vi "ECT in Run on Parametric.vi"(8 "Error In":errorcluster, 9 "ECT Parameters":T1={"MS to Spin Time"=0, "Target Fill Time"=238, "MS to Agitate Time"=0, "MS to Spin before Spin Time "=0, "Adaptive Drain Time"=180, "Coast to 0 Time"=60}, 10 "Option Selection":T2={"Soil Level"=enum."Normal", "Warm Rinse"=enum."Disable", "Fabric Softener"=enum."Disable", "Extra Rinse"=enum."Disable", "Soak"=enum."Level 0", "Stain"=enum."Off", "Spin"=enum."Normal Spin", "Load Size"=enum."Precise Fill", "Dry Load Size"=enum."65535", "Load Type"=enum."Unknown", "Deep Fill"=enum."Off"}, 11 "GEA2 Reference In":refnum<k24>) -> (0 "Error Out":errorcluster, 1 "Pass/Fail?":bool, 2 "Report Text":string, 3 "GEA2 Reference Out":refnum<k24>, 4 "Actual ECT (sec)":u16, 5 "Expected ECT (sec)":u16)   [LabVIEW 2016, in "Centauro.lvlib"]
uses:
  Projects/Centauro.lvlib
  Common/LabVIEW GEA2 Toolkit/LabVIEW_GEA2_Toolkit.lvlibp/type defs/Source_Destination.ctl
  Common/LabVIEW GEA2 Toolkit/LabVIEW_GEA2_Toolkit.lvlibp
  Valew Common/type defs/Encoder Position.ctl
  Common/LabVIEW GEA2 Toolkit/LabVIEW_GEA2_Toolkit.lvlibp/type defs/Data Type.ctl
  Common/LabVIEW GEA2 Toolkit/LabVIEW_GEA2_Toolkit.lvlibp/type defs/ERD Write Data In.ctl
  Valew Common/type defs/UI Buttons.ctl
  Common/LabVIEW GEA2 Toolkit/LabVIEW_GEA2_Toolkit.lvlibp/type defs/ERD Read Data In.ctl
  Q:/Common/DLLs/GEA3/GeaCommunication.dll
  Common/DLLs/GEA3/GeaCommunication.dll
  Controls/Options.ctl
  Controls/ECT Parameters.ctl
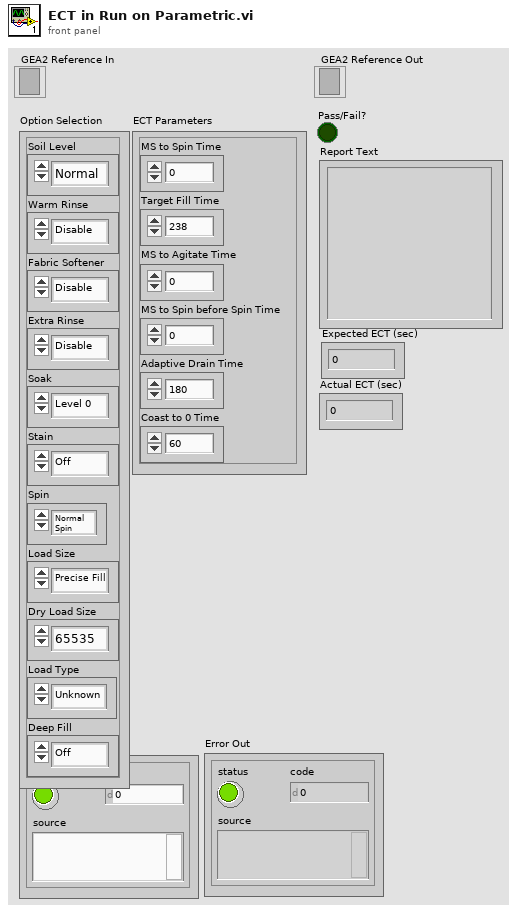
[diagram p1: front panel]
types:
  T1 = typedef "Centauro.lvlib/ECT Parameters.ctl" = cluster{"MS to Spin Time":u16, "Target Fill Time":u16, "MS to Agitate Time":u16, "MS to Spin before Spin Time ":u16, "Adaptive Drain Time":u16, "Coast to 0 Time":u16}
  T2 = typedef "Centauro.lvlib/Options.ctl" = cluster{"Soil Level":enum8{"Ex Light", "Light", "Normal", "Heavy", "Ex Heavy"}, "Warm Rinse":enum8{"Disable", "Enable"}, "Fabric Softener":enum16{"Disable", "Enable"}, "Extra Rinse":enum8{"Disable", "Enable"}, "Soak":enum8{"Level 0", "Level 1", "Level 2", "Level 3", "Level 4"}, "Stain":enum8{"Off", "Tomato", "Wine", "Blood", "Grass", "Dirt"}, "Spin":enum16{"No Spin", "Normal Spin", "More Spin", "Max Spin"}, "Load Size":enum8{"Small", "Medium", "Large", "Super", "Precise Fill", "Super Plus"}, "Dry Load Size":enum16{"128", "256", "384", "5AA", "6A4", "834", "65535"}, "Load Type":enum8{"Unknown", "Cotton", "Synthetic", "Mixed", "Wet", "Low Flow", "Small", "Medium", "Large", "Super", "Super Plus", "Max"}, "Deep Fill":enum8{"Off", "Incremental Fill", "Max Fill"}}
  T3 = typedef "LabVIEW_GEA2_Toolkit.lvlibp/Source_Destination.ctl" = cluster{"Source":u8, "Destination":u8}
  T4 = typedef "LabVIEW_GEA2_Toolkit.lvlibp/ERD Read Data In.ctl" = cluster{"ERD Number":u16, "Data Type":T5}
  T5 = typedef "LabVIEW_GEA2_Toolkit.lvlibp/Data Type.ctl" = enum16{"string", "boolean", "uint8_t", "uint16_t", "uint32_t", "uint64_t", "int8_t", "int16_t", "int32_t", "int64_t"}
  T6 = typedef "Centauro.lvlib/UI Buttons.ctl" = enum16{"Switch Off", "SW201 - My Cycle", "SW202 - Delay Wash", "SW203 - Extra Rinse", "SW204 - Signal / Volume", "SW205 - Spin", "SW206 - Deep Rinse / Fab Soft", "SW207 - Soil", "SW208 - Auto Soak", "SW209 - Temp", "SW210 - Warm Rinse", "SW211 - Deep Fill", "SW212 - Stain Remover", "SW213 - Power", "SW222 - Control Lock", "SW214 - Start / Pause", "SW301 - Start/Pause LE", "SW302 - Option Button LE", "SW201/212 - Bulk Flush"}
  T7 = typedef "LabVIEW_GEA2_Toolkit.lvlibp/ERD Write Data In.ctl" = cluster{"ERD Number":u16, "Data Type":T5, "Data":string}
  T8 = typedef "Centauro.lvlib/Encoder Position.ctl" = enum16{"Position 0", "Position 1", "Position 2", "Position 3", "Position 4", "Position 5", "Position 6", "Position 7", "Position 8", "Position 9", "Position 10", "Position 11", "Position 12", "Position 13", "Clear / Reset"}
  T9 = typedef "LabVIEW_GEA2_Toolkit.lvlibp/ERD Read Data Out.ctl" = cluster{"ERD Number":u16, "Data":string}
  T10 = typedef "Centauro.lvlib/ECT.ctl" = cluster{"MS to Agitate Time":u16, "Adaptive Drain Time":u16, "Coast to 0 Time":u16, "Agitate Time":u16, "Warm Rinse Time":u16, "FS Time":u16, "Ex Rinse Time":u16, "Soak Time":u16, "Stain Time":u16, "Motor Profile ID":u16, "Calculated ECT":u16, "Spin Time":u16}
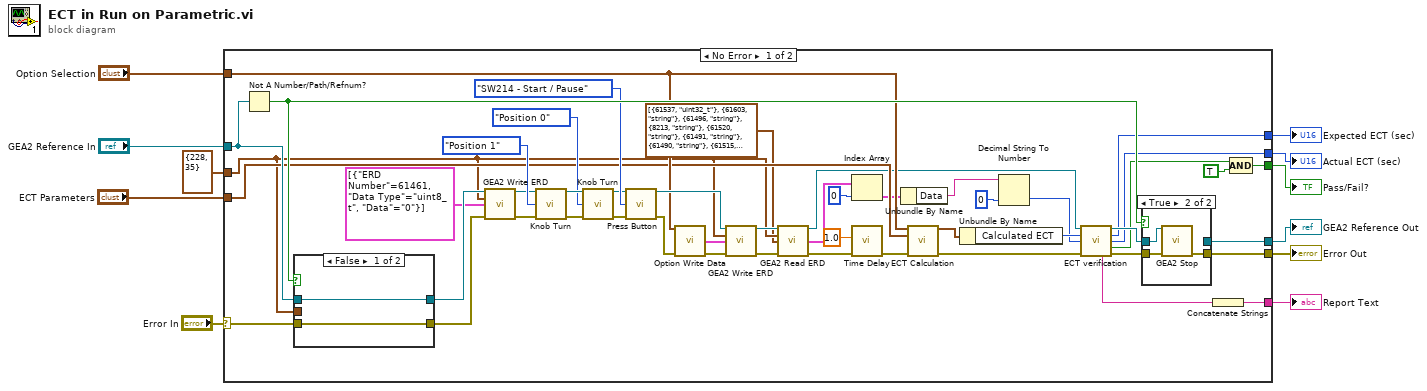
[diagram p0: block diagram]
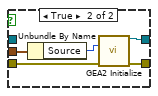
[diagram p3: hidden frame]
diagram:
  n1 = case shown="No Error" "Error In" {
    selector: "Error In" -> [w44 w73]
    tunnel: T3 {"Source"=228, "Destination"=35} ("GEA Inputs") -> [w25 _]
    tunnel: "GEA2 Reference In" -> [w60 w74]
    tunnel: [w35 w74] -> w9
    tunnel: [w59 w73] -> w8
    tunnel: "Option Selection" -> [w43 _]
    tunnel: [w14 _] -> w6
    tunnel: [w58 _] -> w5
    tunnel: "ECT Parameters" -> [w36 _]
    tunnel: [w13 _] -> w2
    tunnel: [w12 _] -> w1
    frame No Error {
      n2 = Not A Number/Path/Refnum?(number/path/refnum=w60) -> (NaN/Path/Refnum?=w48:bool)
      n3 = case shown="False" w48 {
        tunnel: w44 -> [w67 w72]
        tunnel: [w67 w71] -> w53
        tunnel: [w66 w70] -> w52
        tunnel: w25 -> [_ w68]
        tunnel: w60 -> [w66 _]
        frame False {
        }
        frame True {
          n4 = Unbundle By Name(w68) -> ("Source"=w69:u8)
          n5 = call "GEA2 Initialize.vi"("Source Address"=w69, "error in"=w72) -> ("GEA2 Reference Out"=w70:refnum<k24>, "error out"=w71:errorcluster)  [unwired: 11 in, 1 out]
        }
      }
      n6 = call "GEA2 Write ERD.vi"("GEA2 Reference In"=w52, "GEA Inputs"=w25, "Write ERD List"=T7[] [{"ERD Number"=61461, "Data Type"=enum."uint8_t", "Data"="0"}], "Error In"=w53) -> ("GEA2 Reference Out"=w51:refnum<k24>, "Error Out"=w50:errorcluster)  [unwired: 9 in, 1 out]
      n7 = call "Knob Turn.vi"("GEA2 Reference In"=w51, "Button"=Encoder_Position."Position 1", "Error In"=w50) -> ("GEA2 Reference Out"=w56:refnum<k24>, "Error Out"=w55:errorcluster)  [unwired: 11 in]
      n8 = call "Knob Turn.vi"("GEA2 Reference In"=w56, "Button"=Encoder_Position."Position 0", "Error In"=w55) -> ("GEA2 Reference Out"=w42:refnum<k24>, "Error Out"=w41:errorcluster)  [unwired: 11 in]
      n9 = call "Press Button.vi"("GEA2 Reference In"=w42, "Button"=UI_Buttons."SW214 - Start / Pause", "Error In"=w41) -> ("GEA2 Reference Out"=w46:refnum<k24>, "Error Out"=w38:errorcluster)  [unwired: 11 in]
      n10 = call "Option Write Data.vi"("Option Selection"=w43, "Error In"=w38) -> ("appended array"=w40:T7[], "Error Out"=w39:errorcluster)  [unwired: 12 in]
      n11 = call "GEA2 Write ERD.vi"("GEA2 Reference In"=w46, "GEA Inputs"=w25, "Write ERD List"=w40, "Error In"=w39) -> ("GEA2 Reference Out"=w28:refnum<k24>, "Error Out"=w24:errorcluster)  [unwired: 9 in, 1 out]
      n12 = call "GEA2 Read ERD.vi"("GEA2 Reference In"=w28, "GEA Inputs"=w25, "Read ERD List"=T4[] [{"ERD Number"=61537, "Data Type"=enum."uint32_t"}, {"ERD Number"=61603, "Data Type"=enum."string"}, {"ERD Number"=61496, "Data Type"=enum."string"}, {"ERD Number"=8213, "Data Type"=enum."string"}, {"ERD Number"=61520, "Data Type"=enum."string"}, {"ERD Number"=61491, "Data Type"=enum."string"}, {"ERD Number"=61490, "Data Type"=enum."string"}, {"ERD Number"=61515, "Data Type"=enum."string"}, {"ERD Number"=61494, "Data Type"=enum."string"}, {"ERD Number"=61493, "Data Type"=enum."string"}], "Error In"=w24) -> ("GEA2 Reference Out"=w27:refnum<k24>, "ERD Data Out"=w22:T9[], "Error Out"=w26:errorcluster)  [unwired: 8 in, 1 out]
      n13 = Index Array(array=w22, index=0) -> (element=w20:T9)
      n14 = call "Time Delay"("error in (no error)"=w26, "Delay Time (s)"=1.0) -> ("error out"=w45:errorcluster)  [unwired: 9 in]
      n15 = Unbundle By Name(w20) -> ("Data"=w19:string)
      n16 = call "ECT Calculation.vi"("Option Selection"=w43, "ECT Parameters"=w36, "Error In"=w45) -> ("Expected ECT"=w34:T10, "Error Out"=w31:errorcluster)  [unwired: 11 in]
      n17 = Unbundle By Name(w34) -> ("Calculated ECT"=w33:u16)
      n18 = Decimal String To Number(string=w19, default (0L)=0 ("default (0 I32)")) -> (number=w17:i32)  [unwired: 1 in, 1 out]
      n19 = call "ECT verification.vi"(".NET Refnum in"=w27, "Cal ECT (sec)"=w33, "Time remaining (sec)"=w17, "error in"=w31) -> (".NET Refnum out"=w32:refnum<k24>, "Expected ECT (sec)"=w13:u16, "Actual ECT (sec)"=w12:u16, "ECT Pass/Fail"=w29:bool, "Report Text"=w16:string, "error out"=w30:errorcluster)  [unwired: 5 in, 1 out]
      n20 = case shown="True" w48 {
        tunnel: w32 -> [w62 w65]
        tunnel: [w62 _] -> w35
        tunnel: w30 -> [w61 w64]
        tunnel: [w61 w63] -> w59
        frame False {
        }
        frame True {
          n21 = call "GEA2 Stop.vi"("GEA2 Reference In"=w65, "Error In"=w64) -> ("Error Out"=w63:errorcluster)  [unwired: 13 in]
        }
      }
      n22 = Concatenate Strings(w16) -> (w14:string)
      n23 = Compound Arithmetic op=AND(w29, TRUE ("value")) -> (w58:bool)
    }
    frame Error {
    }
  }
  "GEA2 Reference Out" <- w9
  "Error Out" <- w8
  "Report Text" <- w6
  "Pass/Fail?" <- w5
  "Expected ECT (sec)" <- w2
  "Actual ECT (sec)" <- w1
